vi "Monitor Moving Status.vi"(8 "error in (no error)":errorcluster, 9 "YAxis In":refnum<class "iMotion Controller.lvclass">, 10 "X-Axis In":refnum<class "iMotion Controller.lvclass">, 11 "Stage Data Class in":refnum<data-value>) -> (0 "error out":errorcluster, 1 "Y-Axis Out":refnum<class "iMotion Controller.lvclass">, 2 "X-Axis Out":refnum<class "iMotion Controller.lvclass">, 3 "Stage Data Class out":refnum<data-value>)   [LabVIEW 2022 SP3, in "XY Stage Process.lvlib" / "XY Stage Process.lvclass"]
uses:
  XY Stage Process.lvclass
  9c55df22-d0a6-4071-86fa-77dece89c821.vi
  XY Stage Data Class/Moving.ctl
  XY Stage Data Class/XY Stage Data Class.lvclass
  Axis Objects/iMotion Controller/iMotion Controller.lvclass
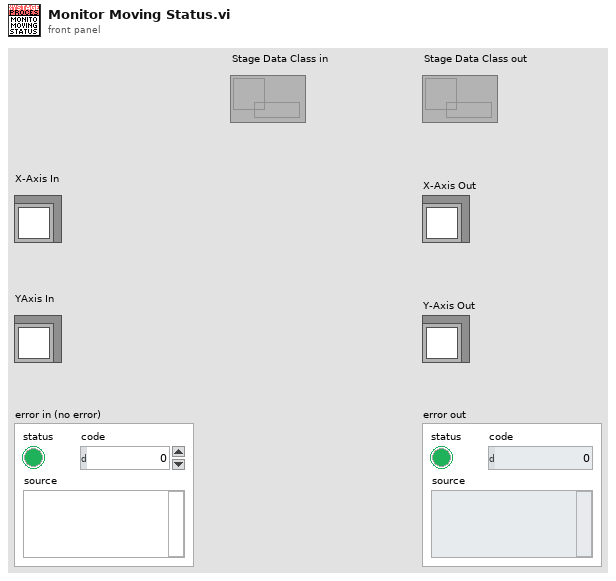
[diagram p1: front panel]
types:
  T1 = typedef "XY Stage Data Class.lvclass/Moving.ctl" = cluster{"X Moving":bool, "Y Moving":bool}
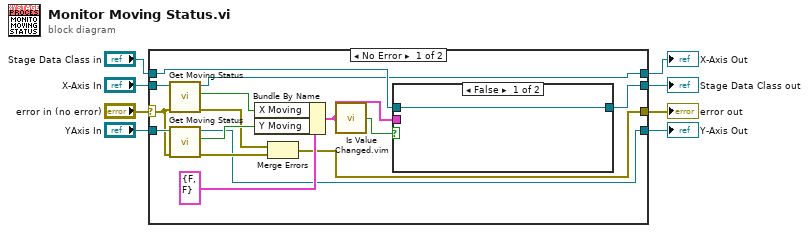
[diagram p0: block diagram]
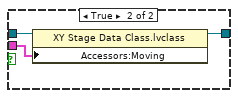
[diagram p2: hidden frame]
diagram:
  n1 = case shown="No Error" "error in (no error)" {
    selector: "error in (no error)" -> [w9 w29]
    tunnel: [w23 w28] -> w8
    tunnel: "YAxis In" -> [w19 w30]
    tunnel: "X-Axis In" -> [w18 w31]
    tunnel: "Stage Data Class in" -> [w17 w28]
    tunnel: [w12 w31] -> w4
    tunnel: [w11 w30] -> w3
    tunnel: [w10 w29] -> w2
    frame No Error {
      n2 = call-dynamic "Get Moving Status.vi"("error in (no error)"=w9, "iMotion Controller in"=w18) -> ("error out"=w13:errorcluster, "Moving"=w21:bool, "iMotion Controller out"=w12:refnum<class "iMotion Controller.lvclass">)  [unwired: 7 in]
      n3 = call-dynamic "Get Moving Status.vi"("error in (no error)"=w9, "iMotion Controller in"=w19) -> ("error out"=w22:errorcluster, "Moving"=w20:bool, "iMotion Controller out"=w11:refnum<class "iMotion Controller.lvclass">)  [unwired: 7 in]
      n4 = Bundle By Name(cluster=T1 {"X Moving"=FALSE, "Y Moving"=FALSE} ("Moving"), "X Moving"=w21, "Y Moving"=w20) -> (w14:T1)
      n5 = Merge Errors(w13, w22) -> (w10:errorcluster)
      n6 = call "Is Value Changed.vim"("value"=w14) -> ("changed or first call?"=w15:bool)
      n7 = case shown="False" w15 {
        tunnel: w14 -> [_ w26]
        tunnel: [w24 w27] -> w23
        tunnel: w17 -> [w24 w25]
        frame False {
        }
        frame True {
          n8 = property class="XY Stage Data Class.lvclass"(reference=w25, "Accessors:Moving"=w26) -> (reference out=w27:refnum<data-value>)  [unwired: 1 in, 1 out]
        }
      }
    }
    frame Error {
    }
  }
  "Stage Data Class out" <- w8
  "X-Axis Out" <- w4
  "Y-Axis Out" <- w3
  "error out" <- w2
